vi "Inverse Dynamics (Trajectory).vi"(0 "serial arm in":refnum<class "NI_Robotics_Serial Robot Arm.lvclass">, 1 "external force":dbl[](array[numeric])=[0.0, 0.0, 0.0, 0.0, 0.0, 0.0], 2 "gravity":dbl[](array[numeric]), 5 "joint position trajectory":dbl[][](array[numeric]), 7 "joint velocity trajectory":dbl[][](array[numeric]), 9 "joint acceleration trajectory":dbl[][](array[numeric]), 11 "error in (no error)":errorcluster) -> (4 "serial arm out":refnum<class "NI_Robotics_Serial Robot Arm.lvclass">, 6 "required torque trajectory":dbl[][](array[numeric]), 15 "error out":errorcluster)   [LabVIEW 2017, in "NI_Kinematics.lvlib"]
doc: "Returns the amount of torque required for the robotic arm to achieve the joint positions, velocities, and accelerations you specify. Wire data to the <B>joint positions</B> input to determine the polymorphic instance to use or manually select the instance.\n\n<B>.m file:</B> rne"
uses:
  <vilib>/robotics/Kinematics/NI_Kinematics.lvlib
  <vilib>/robotics/Kinematics/Robot/NI_Robotics_Serial Robot Arm.lvclass
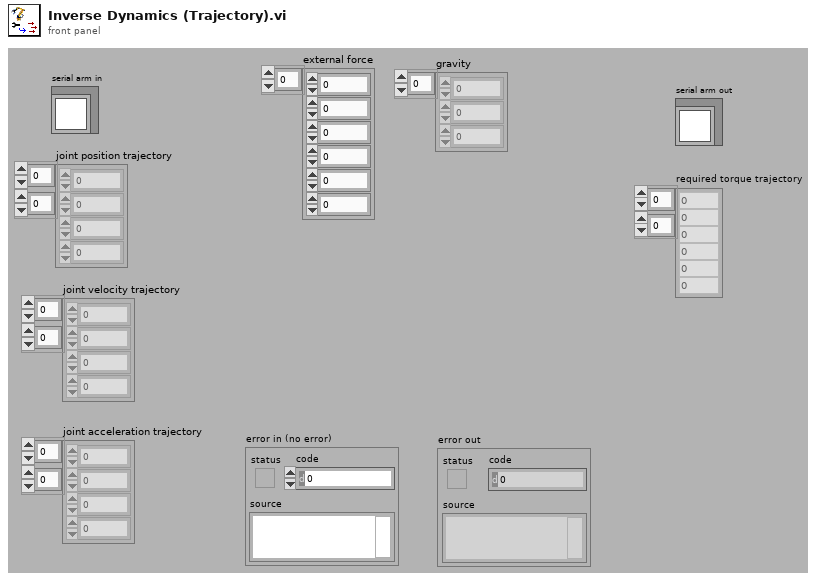
[diagram p1: front panel]
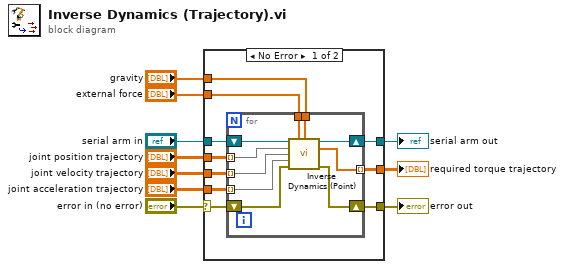
[diagram p0: block diagram]
diagram:
  n1 = case shown="No Error" "error in (no error)" {
    selector: "error in (no error)" -> [w11 w31]
    tunnel: "joint position trajectory" -> [w20 _]
    tunnel: "joint velocity trajectory" -> [w19 _]
    tunnel: "joint acceleration trajectory" -> [w18 _]
    tunnel: [w17 w32] -> w7
    tunnel: [w16 _] -> w6
    tunnel: "external force" -> [w15 _]
    tunnel: "serial arm in" -> [w14 w32]
    tunnel: "gravity" -> [w13 _]
    tunnel: [w12 w31] -> w2
    frame No Error {
      n2 = for {
        tunnel: w20 -> [w28] mode=indexing
        tunnel: w19 -> [w30] mode=indexing
        tunnel: w18 -> [w29] mode=indexing
        tunnel: w15 -> [w26]
        tunnel: w13 -> [w25]
        tunnel: [w23] -> w16 mode=indexing
        shift-right: [w21] -> w12
        shift-left: w11 -> [w22]
        shift-right: [w24] -> w17
        shift-left: w14 -> [w27]
        n3 = call <vilib>:"Inverse Dynamics (Point).vi"("serial arm in"=w27, "external force"=w26, "gravity"=w25, "joint positions"=w28, "joint velocities"=w30, "joint accelerations"=w29, "error in (no error)"=w22) -> ("serial arm out"=w24:refnum<class "NI_Robotics_Serial Robot Arm.lvclass">, "required torques"=w23:dbl[], "error out"=w21:errorcluster)  [unwired: 6 in]
      }
    }
    frame Error {
    }
  }
  "serial arm out" <- w7
  "required torque trajectory" <- w6
  "error out" <- w2
